vi "Check Run Build.vi"(8 "error in (no error)":errorcluster, 10 "Run Instance":refnum<class>, 11 "FPGA Interface in":refnum<class "FPGA Interface.lvclass">) -> (0 "error out":errorcluster, 2 "Correct Build":bool)   [LabVIEW 2026, in "TALOS.lvlib" / "Interfaces.lvlib" / "FPGA Interface.lvclass"]
uses:
  FPGA Interface.lvclass
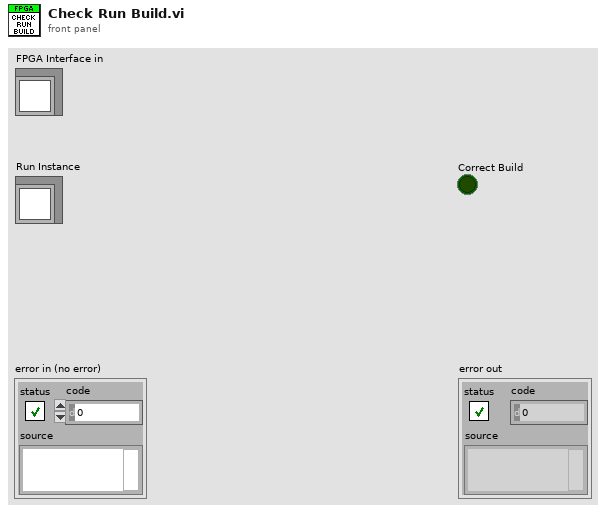
[diagram p1: front panel]
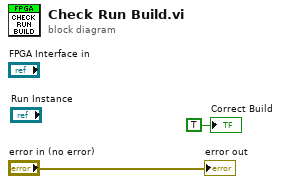
[diagram p0: block diagram]
diagram:
  "error out" <- "error in (no error)"
  "Correct Build" <- TRUE ("Correct Build")
